vi "Main.vi"(11 "Module Admin":refnum<class "Delacor_lib_QMH_Module Admin.lvclass">) -> ()   [LabVIEW 2020, in "UI.lvlib"]
doc: "This template is based off of the Queued Message Handler design pattern and the Queued Message Handler project template that ships with LabVIEW.\n\nThe main difference is that the queue is private to this module and communication between modules is performed via Broadcast and Request events.\n\nRequest events are wrapped in public API methods and are handled in the Event Handling Loop (EHL) of this VI. Any module can register for Broadcast events sent by this module. The EHL generates messages based on user interface actions.\n\nThe Message Handling Loop (MHL) processes messages generated by the EHL, or by other messages. The messages are string values, so new messages can be added easily to the Message Cases case structure in the MHL. Each message cluster can also provide an optional value for Message Data, which is a variant that can be converted to whatever message-specific data is required.\n_____\nBased on Delacor QMH Project Template 5.0.0.82."
uses:
  UI.lvlib
  <vilib>/Delacor/Delacor QMH/Libraries/Module Admin_class/Delacor_lib_QMH_Module Admin.lvclass
  Module Data--cluster.ctl
  Stop Argument--cluster.ctl
  <vilib>/Delacor/Delacor QMH/Libraries/Message Queue_class/Delacor_lib_QMH_Message Queue.lvclass/Delacor_lib_QMH_Message Queue.ctl
  <vilib>/Delacor/Delacor QMH/Libraries/Module Admin_class/Delacor_lib_QMH_Module Admin.lvclass/Delacor_lib_QMH_Module Admin.ctl
  <vilib>/Utility/miscctls.llb/LVPointTypeDef.ctl
  <vilib>/Delacor/Delacor QMH/Libraries/Message Queue_class/Delacor_lib_QMH_Enqueue Message (Single).vi
  <vilib>/Delacor/Delacor QMH/Libraries/Module Admin_class/Delacor_lib_QMH_Get External Launch.vi
  <vilib>/Utility/error.llb/Error Cluster From Error Code.vi
  <vilib>/ErrorRing/Error Ring.xnode
  <vilib>/Delacor/Delacor QMH/Libraries/Message Queue_class/Delacor_lib_QMH_Message Queue.lvclass
  acquisition222/acquisition222.lvlib
panel:
  in  "Stop acquisition":bool
  in  "Start acquisition":bool
  out "error out":errorcluster
  out "Status":string
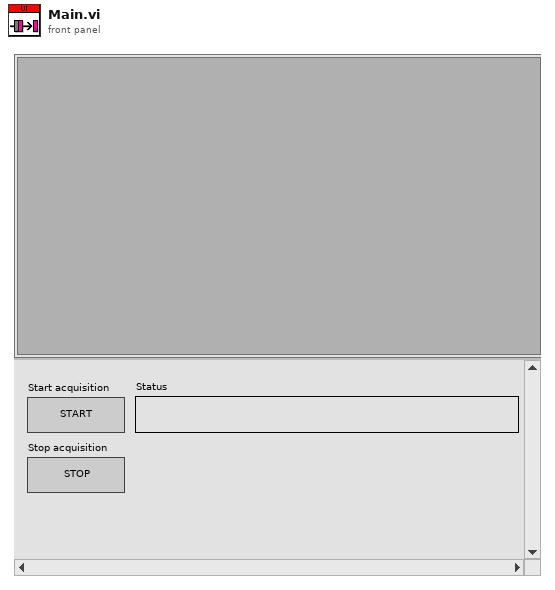
[diagram p1: front panel]
types:
  T1 = typedef "UI.lvlib/Request Events--cluster.ctl" = cluster{"Stop Module":refnum<user-event>, "Show Panel":refnum<user-event>, "Hide Panel":refnum<user-event>, "Get Module Execution Status":refnum<user-event>, "Show Diagram":refnum<user-event>}
  T2 = typedef "acquisition222.lvlib/Broadcast Events--cluster.ctl" = cluster{"Module Did Init":refnum<user-event>, "Status Updated":refnum<user-event>, "Error Reported":refnum<user-event>, "Module Did Stop":refnum<user-event>, "Update Module Execution Status":refnum<user-event>}
  T3 = typedef "UI.lvlib/Module Data--cluster.ctl" = cluster{"Status":string}
  T4 = enum32{"invalid lock state", "Not Locked", "Locked (No Password)", "Password-protected"}
  T5 = typedef "UI.lvlib/Stop Argument--cluster.ctl" = cluster{"Origin":string, "Exit via Stop Module Req?":bool, "Wait for Module to stop?":bool}
  T6 = enum32{"Invalid", "Standard", "Closed", "Hidden", "Minimized", "Maximized"}
  T7 = typedef "LVPointTypeDef.ctl" = cluster{"Horizontal":i16, "Vertical":i16}
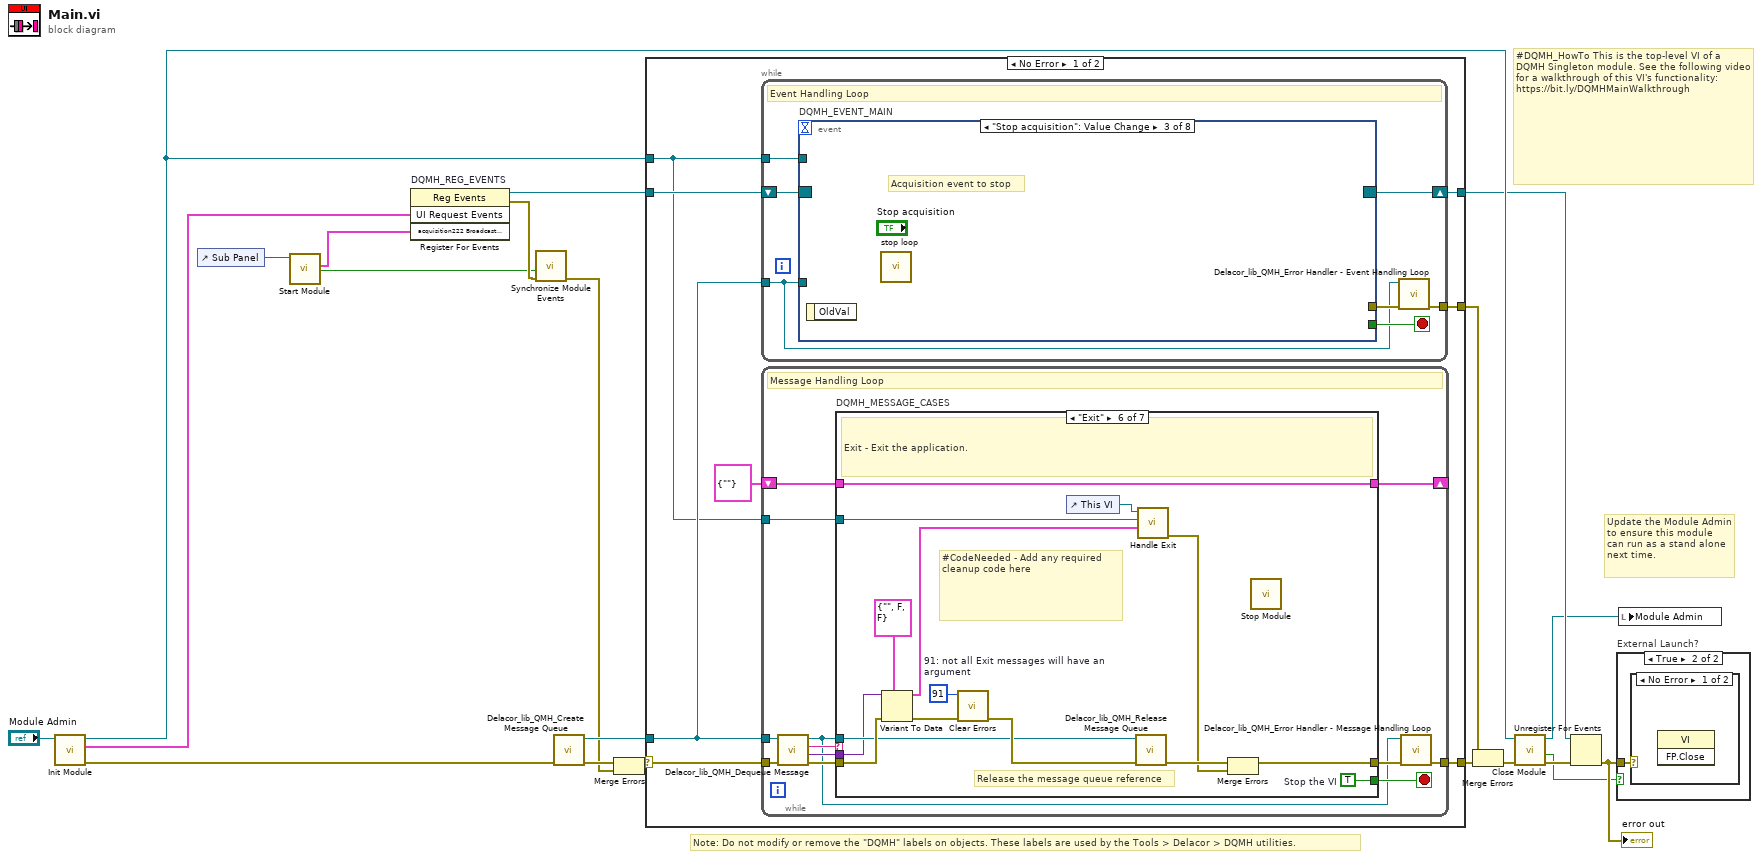
[diagram p0: block diagram]
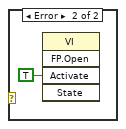
[diagram p3: hidden frame]
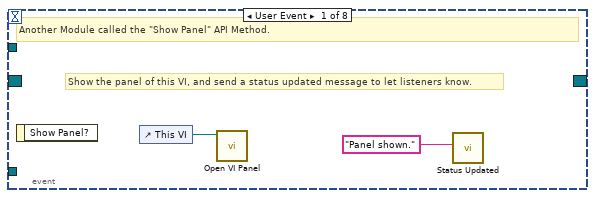
[diagram p4: hidden frame]
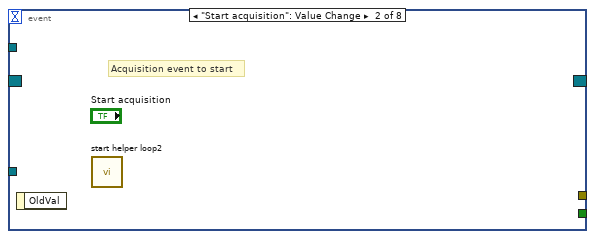
[diagram p5: hidden frame]
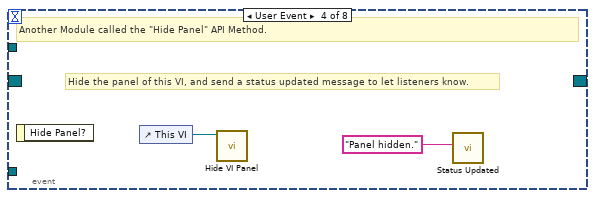
[diagram p6: hidden frame]
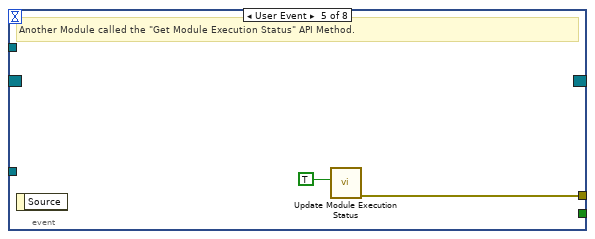
[diagram p7: hidden frame]
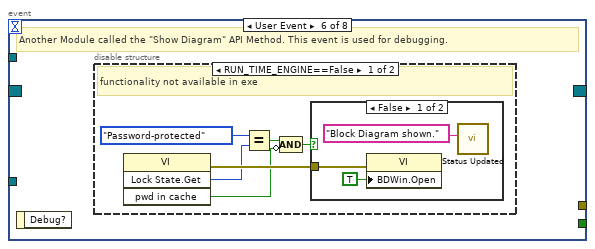
[diagram p8: hidden frame]
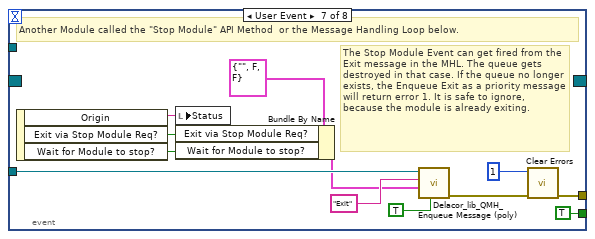
[diagram p11: hidden frame]
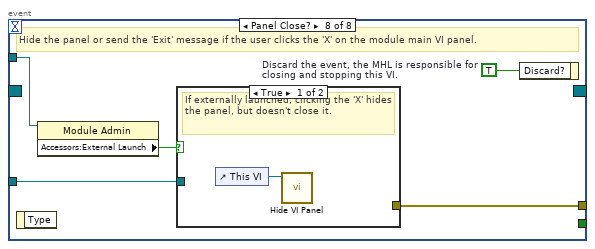
[diagram p12: hidden frame]
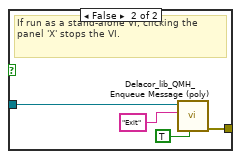
[diagram p13: hidden frame]
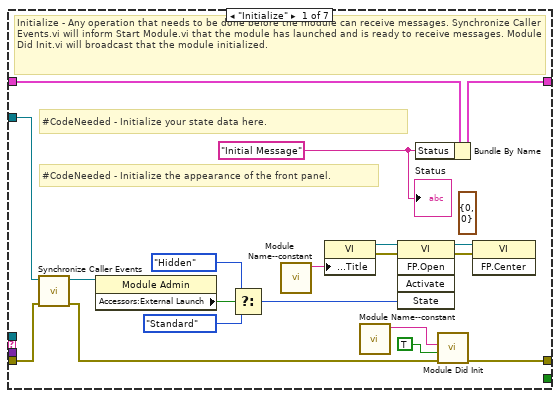
[diagram p14: hidden frame]
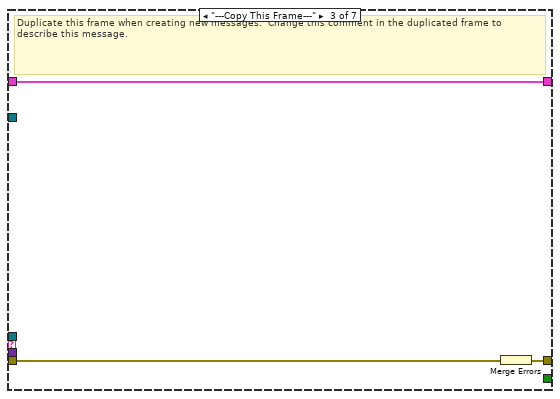
[diagram p16: hidden frame]
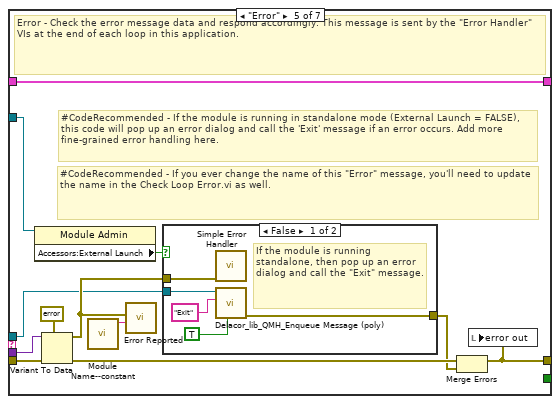
[diagram p18: hidden frame]
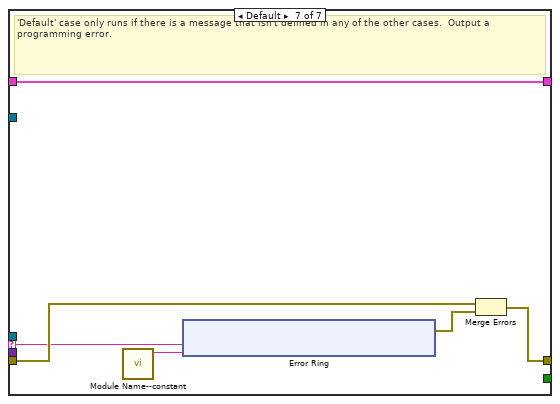
[diagram p20: hidden frame]
diagram:
  # "#DQMH_HowTo This is the top-level VI of a DQMH Singleton module. See the following video for a walkthrough of this VI's functionality: https://bit.ly/DQMHMainWalkthrough"
  # "Note: Do not modify or remove the \"DQMH\" labels on objects. These labels are used by the Tools > Delacor > DQMH utilities."
  # "Update the Module Admin to ensure this module can run as a stand alone next time."
  n1 = call "Init Module.vi"("Singleton Module Admin in"="Module Admin") -> ("error out"=w20:errorcluster, "UI Request Events"=w10:T1, "Singleton Module Admin out"=w13:refnum<class "Delacor_lib_QMH_Module Admin.lvclass">)  [unwired: 8 in]
  n2 = control-ref of="Sub Panel"() -> (w5:refnum<vi>)
  n3 = call "Start Module.vi"("Sub Panel"=w5) -> ("Wait for Event Sync?"=w1:bool, "acquisition222 Broadcast Events"=w4:T2)  [unwired: 7 in, 2 out]
  n4 = register-events "DQMH_REG_EVENTS"(w10, w4) -> (reference out=w11:refnum<event-registration>, error out=w3:errorcluster)  [unwired: 2 in]
  n5 = call "Synchronize Module Events.vi"("error in (no error)"=w3, "Wait for Event Sync?"=w1) -> ("error out"=w2:errorcluster)  [unwired: 9 in]
  n6 = call <vilib>:"Delacor_lib_QMH_Create Message Queue.vi"("error in (no error)"=w20) -> ("error out"=w15:errorcluster, "Message Queue"=w9:refnum<class "Delacor_lib_QMH_Message Queue.lvclass">)  [unwired: 9 in]
  n7 = Merge Errors(w15, w2) -> (w14:errorcluster)
  n8 = case shown="No Error" w14 {
    selector: w14 -> [w27 w160]
    tunnel: [w29 w159] -> w21
    tunnel: [w26 w165] -> w12
    tunnel: w11 -> [w24 w165]
    tunnel: w9 -> [w23 w158]
    tunnel: [w28 _] -> w18
    tunnel: w13 -> [w22 w161]
    frame No Error {
      n9 = while {
        tunnel: w23 -> [w30]
        shift-right: [w33] -> w26
        shift-left: w24 -> [w34]
        tunnel: [w35] -> w28
        tunnel: w22 -> [w31]
        stop <- w32 stop-if-true
        # "Event Handling Loop"
        n10 = event "DQMH_EVENT_MAIN" shown="[2] \"Stop acquisition\": Value Change" {
          selector: w34 -> [_ _ _ _ _ _ _ _]
          dyn-events: [_ _ _ _ _ _ _ _] -> w33
          timeout: _ -> [_ _ _ _ _ _ _ _]
          tunnel: [_ _ _ _ _ _ TRUE ("Discard?") _] -> w32
          tunnel: w30 -> [_ _ _ _ _ _ w59 w66]
          tunnel: [_ _ _ _ w42 _ w62 w68] -> w36
          tunnel: w31 -> [_ _ _ _ _ _ _ w65]
          event User Event {
            # "Show the panel of this VI, and send a status updated message to let listeners know."
            # "Another Module called the \"Show Panel\" API Method."
            n11 = event-data() -> ()  [unwired: 1 in, 1 out]
            n12 = control-ref of="This VI"() -> (w38:refnum<vi>)
            n13 = call "Open VI Panel.vi"("VI"=w38) -> ()  [unwired: 10 in, 1 out]
            n14 = call "Status Updated.vi"("Status"="Panel shown." ("format string")) -> ()  [unwired: 10 in, 1 out]
          }
          event "Start acquisition": Value Change {
            # "Acquisition event to start"
            n15 = event-data() -> ()  [unwired: 1 in, 1 out]
            n16 = call "start helper loop2.vi"() -> ()  [unwired: 11 in, 1 out]
          }
          event "Stop acquisition": Value Change {
            # "Acquisition event to stop"
            n17 = event-data() -> ()  [unwired: 1 in, 1 out]
            n18 = call "stop loop.vi"() -> ()  [unwired: 11 in, 1 out]
          }
          event User Event {
            # "Hide the panel of this VI, and send a status updated message to let listeners know."
            # "Another Module called the \"Hide Panel\" API Method."
            n19 = event-data() -> ()  [unwired: 1 in, 1 out]
            n20 = control-ref of="This VI"() -> (w40:refnum<vi>)
            n21 = call "Hide VI Panel.vi"("VI"=w40) -> ()  [unwired: 10 in, 1 out]
            n22 = call "Status Updated.vi"("Status"="Panel hidden." ("format string")) -> ()  [unwired: 10 in, 1 out]
          }
          event User Event {
            # "Another Module called the \"Get Module Execution Status\" API Method."
            n23 = event-data() -> ()  [unwired: 1 in, 1 out]
            n24 = call "Update Module Execution Status.vi"("Running?"=TRUE) -> ("error out"=w42:errorcluster)  [unwired: 10 in]
          }
          event User Event {
            # "Another Module called the \"Show Diagram\" API Method. This event is used for debugging."
            n25 = event-data() -> ()  [unwired: 1 in, 1 out]
            n26 = disable-structure shown="RUN_TIME_ENGINE==False" {
              frame condition #0 (active) {
                # "functionality not available in exe"
                n27 = invoke class="VI" method="Lock State.Get"() -> (error out=w48:errorcluster, "Get Lock State"=w47:T4, "pwd in cache"=w44:bool)  [unwired: 4 in, 1 out]
                n28 = Equal?(x=T4."Password-protected", y=w47) -> (x = y?=w45:bool)
                n29 = Compound Arithmetic op=AND(w45, invert w44) -> (w43:bool)
                n30 = case shown="False" w43 {
                  tunnel: w48 -> [w51 _]
                  frame False {
                    n31 = property class="VI"(error in=w51, "BDWin.Open"=TRUE ("Block Diagram Window:Open")) -> ()  [unwired: 1 in, 2 out]
                    n32 = call "Status Updated.vi"("Status"="Block Diagram shown." ("format string")) -> ()  [unwired: 10 in, 1 out]
                  }
                  frame True {
                    # "Password-protected VI, and the password is not in the cache. Do not show the diagram."
                  }
                }
              }
              frame condition #1 {
              }
            }
          }
          event User Event {
            # "The Stop Module Event can get fired from the Exit message in the MHL. The queue gets destroyed in that case. If the queue no longer exists, the Enqueue Exit as a priority message will return error 1. It is safe to ignore, because the module is already exiting."
            # "Another Module called the \"Stop Module\" API Method  or the Message Handling Loop below."
            n33 = event-data() -> ("Origin"=w58:string, "Exit via Stop Module Req?"=w54:bool, "Wait for Module to stop?"=w53:bool)  [unwired: 1 in]
            n34 = local write "Status"(w58) -> ()
            n35 = Bundle By Name(cluster=T5 {"Origin"="", "Exit via Stop Module Req?"=FALSE, "Wait for Module to stop?"=FALSE} ("Stop Argument"), "Exit via Stop Module Req?"=w54, "Wait for Module to stop?"=w53) -> (w52:T5)
            n36 = call-poly <vilib>:"Delacor_lib_QMH_Enqueue Message (poly).vi"("Priority Message? (F)"=TRUE, "Message Data"=w52, "Message"="Exit", "Message Queue in"=w59) -> ("error out"=w63:errorcluster)  [unwired: 6 in, 1 out]
            n37 = call <vilib>:"Clear Errors.vi"("error in (no error)"=w63, "specific error code to clear (0: all)"=1) -> ("error out"=w62:errorcluster)  [unwired: 4 in, 1 out]
          }
          event Panel Close? {
            w67 = TRUE  # Discard the event, the MHL is responsible for closing and stopping this VI.
            # "Hide the panel or send the 'Exit' message if the user clicks the 'X' on the module main VI panel."
            n38 = event-data() -> ()  [unwired: 1 in, 1 out]
            n39 = property class="Module Admin"(reference=w65) -> ("Accessors:External Launch"=w64:bool)  [unwired: 1 in, 2 out]
            n40 = case shown="True" w64 {
              tunnel: w66 -> [_ w72]
              tunnel: [_ w73] -> w68
              frame True {
                # "If externally launched, clicking the 'X' hides the panel, but doesn't close it."
                n41 = control-ref of="This VI"() -> (w69:refnum<vi>)
                n42 = call "Hide VI Panel.vi"("VI"=w69) -> ()  [unwired: 10 in, 1 out]
              }
              frame False {
                # "If run as a stand-alone VI, clicking the panel 'X' stops the VI."
                n43 = call-poly <vilib>:"Delacor_lib_QMH_Enqueue Message (poly).vi"("Priority Message? (F)"=TRUE, "Message"="Exit", "Message Queue in"=w72) -> ("error out"=w73:errorcluster)  [unwired: 7 in, 1 out]
              }
            }
            n44 = event-data("Discard?"=w67) -> ()  [unwired: 1 in, 1 out]
          }
        }
        n45 = call-dynamic "Delacor_lib_QMH_Error Handler - Event Handling Loop.vi"("error in (no error)"=w36, "Message Queue in"=w30) -> ("dup error in"=w35:errorcluster)  [unwired: 8 in, 1 out]
      }
      n46 = while {
        tunnel: w23 -> [w76]
        shift-right: [w80] -> _
        shift-left: T3 {"Status"=""} ("Data Cluster") -> [w81]
        tunnel: w27 -> [w84]
        tunnel: [w82] -> w29
        tunnel: w22 -> [w74]
        stop <- w79 stop-if-true
        # "Message Handling Loop"
        n47 = call-dynamic "Delacor_lib_QMH_Dequeue Message.vi"("error in (no error)"=w84, "Message Queue in"=w76) -> ("error out"=w83:errorcluster, "Message Data"=w77:variant, "Message"=w78:string, "Message Queue out"=w75:refnum<class "Delacor_lib_QMH_Message Queue.lvclass">)  [unwired: 6 in]
        n48 = case "DQMH_MESSAGE_CASES" shown="\"Exit\"" w78 {
          selector: w78 -> [_ _ _ _ _ _ w145]
          tunnel: w75 -> [_ _ _ _ w115 w137 _]
          tunnel: w83 -> [w102 w106 w109 w111 w122 w143 w147]
          tunnel: [w100 w106 w108 w111 w118 w140 w148] -> w85
          tunnel: w81 -> [w91 w105 w107 w110 w117 w136 w146]
          tunnel: [w90 w105 w107 w110 w117 w136 w146] -> w80
          tunnel: [_ _ _ _ _ w135 _] -> w79
          tunnel: w77 -> [_ _ _ _ w116 w134 _]
          tunnel: w74 -> [w92 _ _ _ w114 w129 _]
          frame "Initialize" {
            (unwired) T7 {"Horizontal"=0, "Vertical"=0} ("Origin")
            w86 = "Initial Message" ("Initial Message")
            # "#CodeNeeded - Initialize the appearance of the front panel."
            # "#CodeNeeded - Initialize your state data here."
            # "Initialize - Any operation that needs to be done before the module can receive messages. Synchronize Caller Events.vi will inform Start Module.vi that the module has launched and is ready to receive messages. Module Did Init.vi will broadcast that the module initialized."
            n49 = call "Synchronize Caller Events.vi"("error in (no error)"=w102, "Singleton Module Admin in"=w92) -> ("error out"=w101:errorcluster, "Singleton Module Admin out"=w87:refnum<class "Delacor_lib_QMH_Module Admin.lvclass">)  [unwired: 8 in]
            n50 = property class="Module Admin"(reference=w87) -> ("Accessors:External Launch"=w96:bool)  [unwired: 1 in, 2 out]
            n51 = Select(t=T6."Hidden" ("State"), s=w96, f=T6."Standard" ("State")) -> (s? t:f=w93:T6)
            n52 = call "Module Name--constant.vi"() -> ("Module Name"=w99:string)  [unwired: 11 in]
            n53 = property class="VI"("Front Panel.Title"=w99) -> (reference out=w98:refnum<vi>, error out=w104:errorcluster)  [unwired: 2 in]
            n54 = call "Module Name--constant.vi"() -> ("Module Name"=w88:string)  [unwired: 11 in]
            n55 = invoke class="VI" method="FP.Open"(reference=w98, error in=w104, "State"=w93) -> (reference out=w97:refnum<vi>, error out=w103:errorcluster)  [unwired: 2 in, 3 out]
            n56 = Bundle By Name(cluster=w91, "Status"=w86) -> (w90:T3)
            n57 = call "Module Did Init.vi"("error in (no error)"=w101, "Initialized?"=TRUE, "Origin"=w88) -> ("error out"=w100:errorcluster)  [unwired: 8 in]
            n58 = invoke class="VI" method="FP.Center"(reference=w97, error in=w103) -> ()  [unwired: 1 in, 3 out]
            "Status" <- w86
          }
          frame "--- Module Specific ---" {
            # "Separator -- The following cases handle messages specific to this Module."
          }
          frame "---Copy This Frame---" {
            # "Duplicate this frame when creating new messages.  Change this comment in the duplicated frame to describe this message."
            n59 = Merge Errors(w109) -> (w108:errorcluster)
          }
          frame "--- Exit and Error Handling---" {
            # "Separator - The following cases handle errors and exit messages."
          }
          frame "Error" {
            # "#CodeRecommended - If you ever change the name of this \"Error\" message, you'll need to update the name in the Check Loop Error.vi as well."
            # "#CodeRecommended - If the module is running in standalone mode (External Launch = FALSE), this code will pop up an error dialog and call the 'Exit' message if an error occurs. Add more fine-grained error handling here."
            # "Error - Check the error message data and respond accordingly. This message is sent by the \"Error Handler\" VIs at the end of each loop in this application."
            n60 = property class="Module Admin"(reference=w114) -> ("Accessors:External Launch"=w113:bool)  [unwired: 1 in, 2 out]
            n61 = Variant To Data(error in=w122, type=errorcluster {"status"=FALSE, "code"=0, "source"=""} ("error constant"), Variant=w116) -> (data=w123:errorcluster, error out=w120:errorcluster)
            n62 = call "Module Name--constant.vi"() -> ("Module Name"=w112:string)  [unwired: 11 in]
            n63 = call "Error Reported.vi"("Additional Information"=w112, "Error"=w123) -> ()  [unwired: 9 in, 1 out]
            n64 = case shown="False" w113 {
              tunnel: [w128 _] -> w119
              tunnel: w115 -> [w126 _]
              tunnel: w123 -> [w127 _]
              frame False {
                # "If the module is running standalone, then pop up an error dialog and call the \"Exit\" message."
                n65 = call <vilib>:"Simple Error Handler.vi"("error in (no error)"=w127) -> ()  [unwired: 4 in, 5 out]
                n66 = call-poly <vilib>:"Delacor_lib_QMH_Enqueue Message (poly).vi"("Priority Message? (F)"=TRUE, "Message"="Exit", "Message Queue in"=w126) -> ("error out"=w128:errorcluster)  [unwired: 7 in, 1 out]
              }
              frame True {
                # "If the module was launched externally, calling the Error Reported broadcast VI is the only action performed by the \"Error\" message. The module's caller can then process the error appropriately."
              }
            }
            n67 = Merge Errors(w120, w119) -> (w118:errorcluster)
            n68 = local write "error out"(w118) -> ()
          }
          frame "Exit" {
            w133 = 91  # 91: not all Exit messages will have an argument
            w135 = TRUE  # Stop the VI
            # "Release the message queue reference"
            # "#CodeNeeded - Add any required cleanup code here"
            # "Exit - Exit the application."
            n69 = Variant To Data(error in=w143, type=T5 {"Origin"="", "Exit via Stop Module Req?"=FALSE, "Wait for Module to stop?"=FALSE} ("Stop Argument"), Variant=w134) -> (data=w131:T5, error out=w139:errorcluster)
            n70 = call <vilib>:"Clear Errors.vi"("error in (no error)"=w139, "specific error code to clear (0: all)"=w133) -> ("error out"=w142:errorcluster)  [unwired: 4 in, 1 out]
            n71 = control-ref of="This VI"() -> (w130:refnum<vi>)
            n72 = call-dynamic "Delacor_lib_QMH_Release Message Queue.vi"("error in (no error)"=w142, "Message Queue"=w137) -> ("error out"=w141:errorcluster)  [unwired: 9 in]
            n73 = call "Handle Exit.vi"("Stop Argument"=w131, "Admin in"=w129, "VI reference"=w130) -> ("error out"=w138:errorcluster)  [unwired: 7 in, 1 out]
            n74 = Merge Errors(w141, w138) -> (w140:errorcluster)
            n75 = call "Stop Module.vi"() -> ()  [unwired: 11 in, 1 out]
          }
          frame Default {
            # "'Default' case only runs if there is a message that isn't defined in any of the other cases.  Output a programming error."
            n76 = call "Module Name--constant.vi"() -> ("Module Name"=w144:string)  [unwired: 11 in]
            n77 = xnode "Error Ring"("parameter 0"=w145, "parameter 1"=w144) -> ("error out"=w149:errorcluster)
            n78 = Merge Errors(w147, w149) -> (w148:errorcluster)
          }
        }
        n79 = call-dynamic "Delacor_lib_QMH_Error Handler - Message Handling Loop.vi"("error in (no error)"=w85, "Message Queue in"=w75) -> ("dup error in"=w82:errorcluster)  [unwired: 8 in, 1 out]
      }
    }
    frame Error {
      # "Synchronize Caller Events.vi will inform Start Module.vi that the module has launched and will let the code calling Start Module.vi register for broadcasts and would permit the caller receive the broadcast that an error occurred at launch time."
      n80 = call-dynamic "Delacor_lib_QMH_Release Message Queue.vi"("error in (no error)"=w160, "Message Queue"=w158) -> ("error out"=w159:errorcluster)  [unwired: 9 in]
      n81 = call "Synchronize Caller Events.vi"("Singleton Module Admin in"=w161) -> ("error out"=w166:errorcluster)  [unwired: 9 in, 1 out]
      n82 = call "Module Name--constant.vi"() -> ("Module Name"=w164:string)  [unwired: 11 in]
      n83 = Format Into String(format string="An error occurred during initialization. %s is no longer running.", w164) -> (resulting string=w162:string)  [unwired: 2 in, 1 out]
      n84 = Merge Errors(w159, w166) -> (w167:errorcluster)
      n85 = call "Error Reported.vi"("Additional Information"=w162, "Error"=w167) -> ()  [unwired: 9 in, 1 out]
    }
  }
  n86 = Merge Errors(w18, w21) -> (w17:errorcluster)
  n87 = call "Close Module.vi"("error in (no error)"=w17, "Module Admin in"=w13) -> ("error out"=w19:errorcluster, "External Launch"=w6:bool, "Module Admin out"=w7:refnum<class "Delacor_lib_QMH_Module Admin.lvclass">)  [unwired: 7 in]
  n88 = Unregister For Events(event registration refnum=w12, error in=w19) -> (error out=w16:errorcluster)
  "error out" <- w16
  n89 = case "External Launch?" shown="True" w6 {
    tunnel: w16 -> [_ w168]
    frame False {
    }
    frame True {
      n90 = case shown="No Error" w168 {
        frame No Error {
          n91 = invoke class="VI" method="FP.Close"() -> ()  [unwired: 3 in, 3 out]
        }
        frame Error {
          n92 = invoke class="VI" method="FP.Open"("Activate"=TRUE ("Activate?")) -> ()  [unwired: 4 in, 5 out]
        }
      }
    }
  }
  n93 = local write "Module Admin"(w7) -> ()
